vi "压装试验判定.vi"(7 "Result":refnum<vi>, 10 "判定参数":T1, 11 "XY曲线":cluster{"X":dbl[], "Y":dbl[]}[](array[cluster])) -> (2 "判定项长度":i32, 3 "OK？":bool)   [LabVIEW 2020]
panel:
  out "正向平均值":dbl
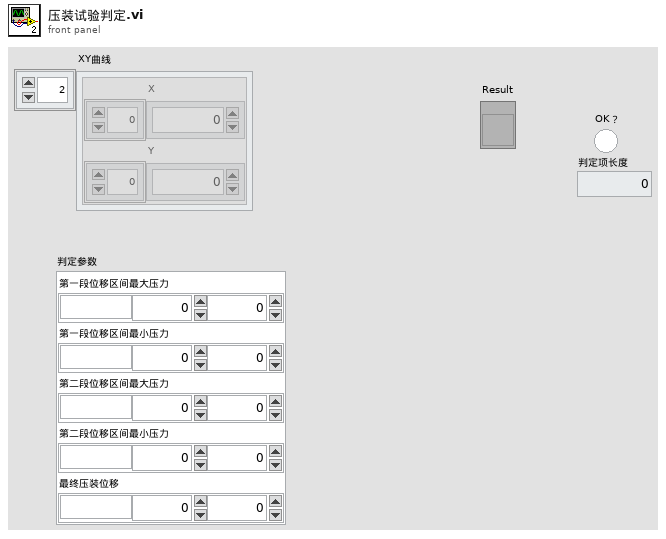
[diagram p1: front panel]
types:
  T1 = cluster{"第一段位移区间最大压力":cluster{"单位":string, "下限":dbl, "上限":dbl}, "第一段位移区间最小压力":cluster{"单位":string, "下限":dbl, "上限":dbl}, "第二段位移区间最大压力":cluster{"单位":string, "下限":dbl, "上限":dbl}, "第二段位移区间最小压力":cluster{"单位":string, "下限":dbl, "上限":dbl}, "最终压装位移":cluster{"单位":string, "下限":dbl, "上限":dbl}}
  T2 = cluster{"1位移":cluster{"单位":string, "下限":dbl, "上限":dbl}, "1压力":cluster{"单位":string, "下限":dbl, "上限":dbl}, "2位移":cluster{"单位":string, "下限":dbl, "上限":dbl}, "2压力":cluster{"单位":string, "下限":dbl, "上限":dbl}}
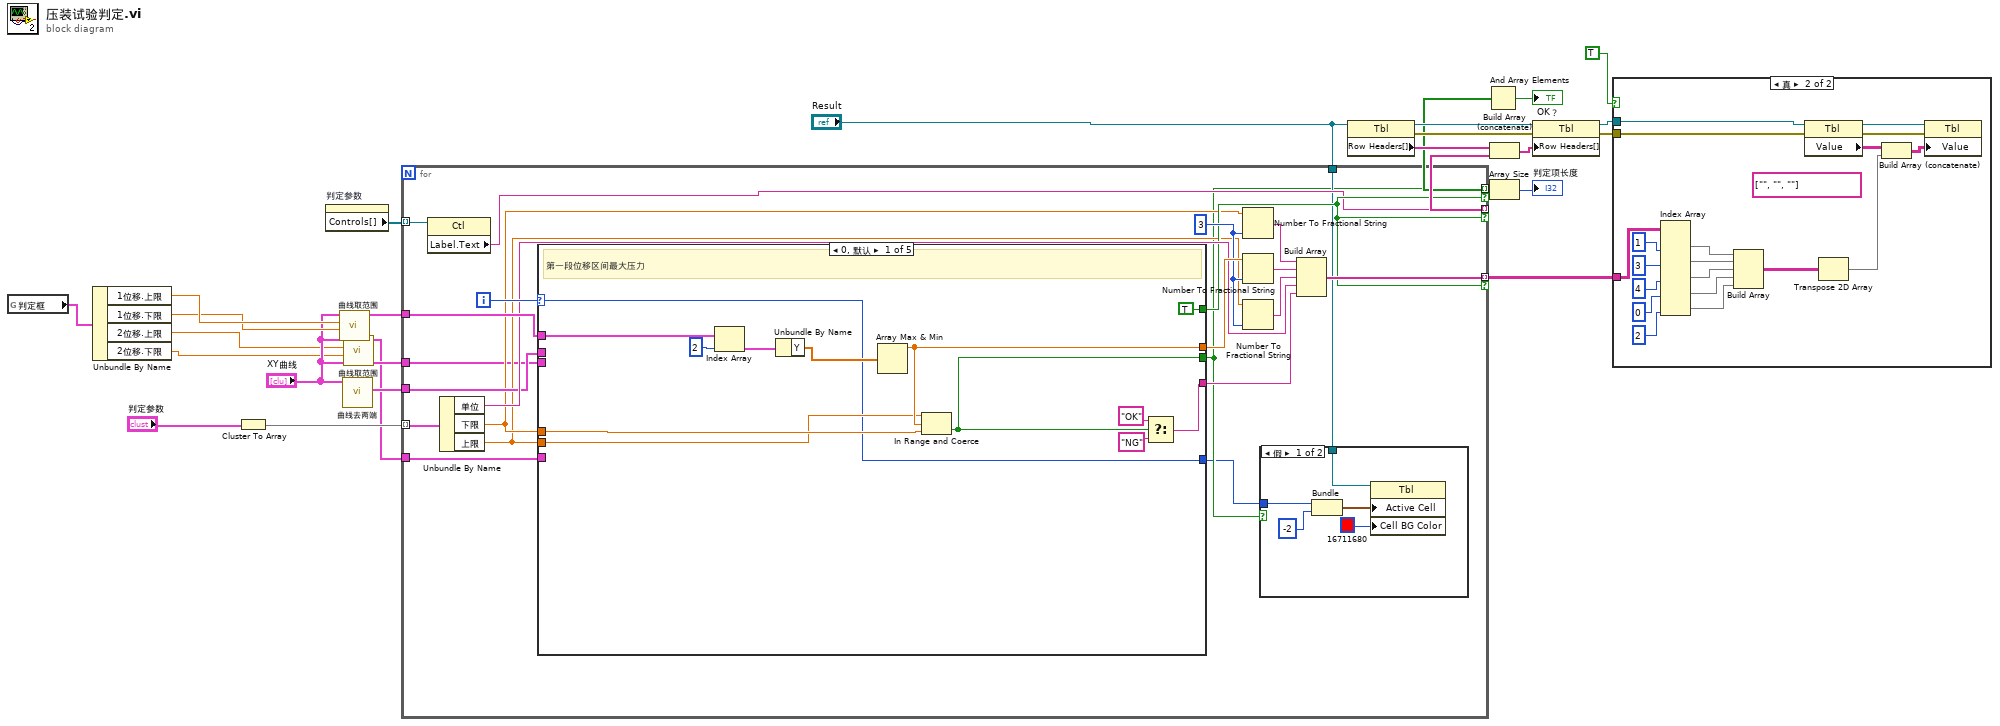
[diagram p0: block diagram]
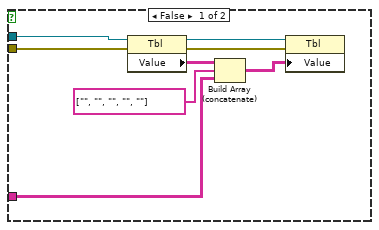
[diagram p2: hidden frame]
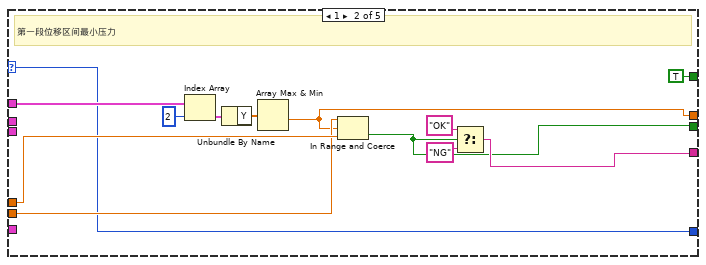
[diagram p4: hidden frame]
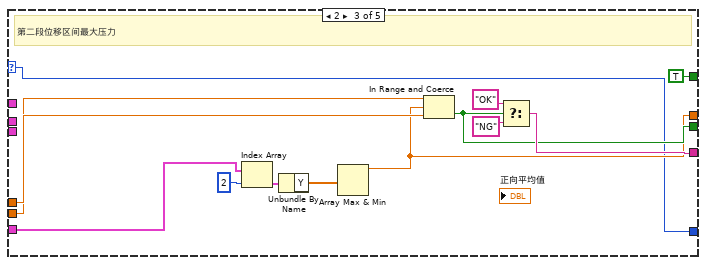
[diagram p5: hidden frame]
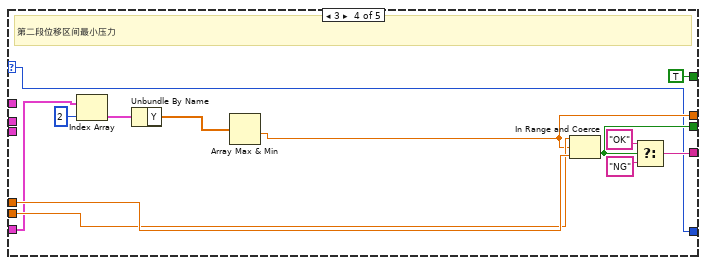
[diagram p6: hidden frame]
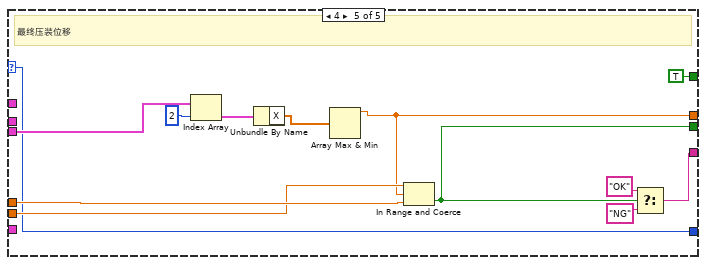
[diagram p7: hidden frame]
diagram:
  n1 = global read "判定参数.vi" "判定框"() -> (w6:T2)
  n2 = Unbundle By Name(w6) -> ("1位移.上限"=w8:dbl, "1位移.下限"=w7:dbl, "2位移.上限"=w4:dbl, "2位移.下限"=w3:dbl)
  n3 = Cluster To Array(cluster="判定参数") -> (array=w25:cluster{"单位":string, "下限":dbl, "上限":dbl}[])
  n4 = property on="判定参数" class="Clust (严格)"() -> ("Controls[]"=w15:refnum<vi>[])  [unwired: 2 in, 2 out]
  n5 = call "曲线取范围.vi"("下限"=w7, "上限"=w8, "曲线In"="XY曲线") -> ("曲线Out"=w10:cluster{"X":dbl[], "Y":dbl[]}[])  [unwired: 8 in]
  n6 = call "曲线去两端.vi"("曲线In"="XY曲线") -> ("启动曲线"=w11:cluster{"X":dbl[], "Y":dbl[]}[])  [unwired: 9 in, 1 out]
  n7 = call "曲线取范围.vi"("下限"=w3, "上限"=w4, "曲线In"="XY曲线") -> ("曲线Out"=w2:cluster{"X":dbl[], "Y":dbl[]}[])  [unwired: 8 in]
  n8 = for {
    tunnel: w25 -> [w47] mode=indexing
    tunnel: w15 -> [w45] mode=indexing
    tunnel: w10 -> [w43]
    tunnel: [w27] -> w13 mode=indexing if=w35
    tunnel: [w36] -> w16 mode=indexing if=w35
    tunnel: [w31] -> w18 mode=indexing if=w35
    tunnel: w11 -> [w34]
    tunnel: "XY曲线" -> [w30]
    tunnel: w2 -> [w29]
    tunnel: "Result" -> [w28]
    i -> [w46]
    w42 = i16 3 ("精度(6)")
    n9 = property class="Ctl"(reference=w45) -> ("Label.Text"=w31:string)  [unwired: 1 in, 2 out]
    n10 = Unbundle By Name(w47) -> ("单位"=w37:string, "下限"=w33:dbl, "上限"=w32:dbl)
    n11 = case shown="0, 默认" w46 {
      selector: w46 -> [w53 w66 w79 w92 w105]
      tunnel: [w62 w69 w80 w93 w106] -> w44
      tunnel: w43 -> [w65 w78 _ _ _]
      tunnel: [w59 w74 w89 w102 w113] -> w38
      tunnel: [w58 w73 w88 w101 w112] -> w27
      tunnel: w33 -> [w57 w72 w87 w100 w111]
      tunnel: w32 -> [w56 w71 w86 w99 w110]
      tunnel: [TRUE TRUE TRUE TRUE TRUE] -> w35
      tunnel: w34 -> [_ _ _ _ _]
      tunnel: w30 -> [_ _ _ _ w107]
      tunnel: w29 -> [_ _ w82 w94 _]
      tunnel: [w53 w66 w79 w92 w105] -> w26
      frame 0, Default {
        # "第一段位移区间最大压力"
        n12 = Index Array(array=w65, index=2 ("索引")) -> (element=w63:cluster{"X":dbl[], "Y":dbl[]})
        n13 = Unbundle By Name(w63) -> ("Y"=w54:dbl[])
        n14 = Array Max & Min(array=w54) -> (max value=w62:dbl)  [unwired: 3 out]
        n15 = In Range and Coerce(upper limit=w56, x=w62, lower limit=w57) -> (In Range?=w58:bool)  [unwired: 1 out]
        n16 = Select(t="OK", s=w58, f="NG") -> (s? t:f=w59:string)
      }
      frame 1 {
        # "第一段位移区间最小压力"
        n17 = Index Array(array=w78, index=2 ("索引")) -> (element=w77:cluster{"X":dbl[], "Y":dbl[]})
        n18 = Unbundle By Name(w77) -> ("Y"=w68:dbl[])
        n19 = Array Max & Min(array=w68) -> (min value=w69:dbl)  [unwired: 3 out]
        n20 = In Range and Coerce(upper limit=w71, x=w69, lower limit=w72) -> (In Range?=w73:bool)  [unwired: 1 out]
        n21 = Select(t="OK", s=w73, f="NG") -> (s? t:f=w74:string)
      }
      frame 2 {
        # "第二段位移区间最大压力"
        n22 = Index Array(array=w82, index=2 ("索引")) -> (element=w84:cluster{"X":dbl[], "Y":dbl[]})
        n23 = Unbundle By Name(w84) -> ("Y"=w81:dbl[])
        n24 = Array Max & Min(array=w81) -> (max value=w80:dbl)  [unwired: 3 out]
        n25 = In Range and Coerce(upper limit=w86, x=w80, lower limit=w87) -> (In Range?=w88:bool)  [unwired: 1 out]
        n26 = Select(t="OK", s=w88, f="NG") -> (s? t:f=w89:string)
      }
      frame 3 {
        # "第二段位移区间最小压力"
        n27 = Index Array(array=w94, index=2 ("索引")) -> (element=w97:cluster{"X":dbl[], "Y":dbl[]})
        n28 = Unbundle By Name(w97) -> ("Y"=w95:dbl[])
        n29 = Array Max & Min(array=w95) -> (min value=w93:dbl)  [unwired: 3 out]
        n30 = In Range and Coerce(upper limit=w99, x=w93, lower limit=w100) -> (In Range?=w101:bool)  [unwired: 1 out]
        n31 = Select(t="OK", s=w101, f="NG") -> (s? t:f=w102:string)
      }
      frame 4 {
        # "最终压装位移"
        n32 = Index Array(array=w107, index=2 ("索引")) -> (element=w116:cluster{"X":dbl[], "Y":dbl[]})
        n33 = Unbundle By Name(w116) -> ("X"=w108:dbl[])
        n34 = Array Max & Min(array=w108) -> (max value=w106:dbl)  [unwired: 3 out]
        n35 = In Range and Coerce(upper limit=w110, x=w106, lower limit=w111) -> (In Range?=w112:bool)  [unwired: 1 out]
        n36 = Select(t="OK", s=w112, f="NG") -> (s? t:f=w113:string)
      }
    }
    n37 = Number To Fractional String(number=w33, precision (6)=w42) -> (F-format string=w41:string)  [unwired: 2 in]
    n38 = Number To Fractional String(number=w44, precision (6)=w42) -> (F-format string=w40:string)  [unwired: 2 in]
    n39 = Number To Fractional String(number=w32, precision (6)=w42) -> (F-format string=w39:string)  [unwired: 2 in]
    n40 = case shown="假" w27 {
      tunnel: w28 -> [w52 _]
      tunnel: w26 -> [w48 _]
      frame False {
        n41 = Bundle(w48, "索引"=-2) -> (w49:cluster{i32, "索引":i32})  [unwired: 1 in]
        n42 = property class="Tbl"(reference=w52, "Active Cell"=w49, "Cell BG Color"=u32 16711680 ("活动单元格:单元格背景色")) -> ()  [unwired: 1 in, 2 out]
      }
      frame True {
      }
    }
    n43 = Build Array(w41, w40, w39, w37, w38) -> (w36:string[])
  }
  n44 = property class="Tbl"(reference="Result") -> (reference out=w20:refnum<vi>, error out=w23:errorcluster, "Row Headers[]"=w17:string[])  [unwired: 1 in]
  n45 = And Array Elements(Boolean array=w13) -> (logical AND=→"OK？":bool)
  n46 = Build Array (concatenate)(w17, w18) -> (w19:string[])
  n47 = Array Size(array=w13) -> (size(s)=→"判定项长度":i32)
  n48 = property class="Tbl"(reference=w20, error in=w23, "Row Headers[]"=w19) -> (reference out=w21:refnum<vi>, error out=w22:errorcluster)
  n49 = case shown="真" TRUE {
    tunnel: w22 -> [w123 w142]
    tunnel: w21 -> [w120 w139]
    tunnel: w16 -> [w119 w138]
    frame False {
      n50 = property class="Tbl"(reference=w120, error in=w123) -> (reference out=w121:refnum<vi>, error out=w122:errorcluster, "Value"=w124:string[][])
      n51 = Build Array (concatenate)(w124, string[] ["", "", "", "", ""], w119) -> (w125:string[][])
      n52 = property class="Tbl"(reference=w121, error in=w122, "Value"=w125) -> ()  [unwired: 2 out]
    }
    frame True {
      (unwired) string[] ["", "", ""]
      n53 = Index Array(array=w138, index (col) #1=1 ("禁用的索引 (列)"), index (col) #2=3 ("索引 (列)"), index (col) #3=4 ("索引 (列)"), index (col) #4=0 ("索引 (列)"), index (col) #5=2 ("索引 (列)")) -> (element #1=w134:string[], element #2=w133:string[], element #3=w132:string[], element #4=w127:string[], element #5=w126:string[])  [unwired: 5 in]
      n54 = Build Array(w134, w133, w132, w127, w126) -> (w131:string[][])
      n55 = property class="Tbl"(reference=w139, error in=w142) -> (reference out=w140:refnum<vi>, error out=w141:errorcluster, "Value"=w143:string[][])
      n56 = Transpose 2D Array(2D array=w131) -> (transposed array=w130:string[][])
      n57 = Build Array (concatenate)(w143, w130) -> (w144:string[][])
      n58 = property class="Tbl"(reference=w140, error in=w141, "Value"=w144) -> ()  [unwired: 2 out]
    }
  }
